vi "Encapsulate TCP Message.vi"(5 "source_id":u32, 7 "target_id":u32, 8 "error in (no error)":errorcluster, 9 "type_id":u32, 10 "Encapsulated Msg":refnum<class "Message.lvclass">) -> (0 "error out":errorcluster, 2 "TCP Payload":string)   [LabVIEW 2020, in "Vecto.lvlib"]
uses:
  Vecto.lvlib
  <vilib>/IlluminatedG/IG Protoc/LV-Proto/Message/Message.lvclass
  SequenceCountService/SequenceCountService.lvclass
  proto/TcpPayload/Data.ctl
  proto/TcpPayload/TcpPayload.lvlib
panel:
  in  "SequenceCountService":refnum<class "SequenceCountService.lvclass">
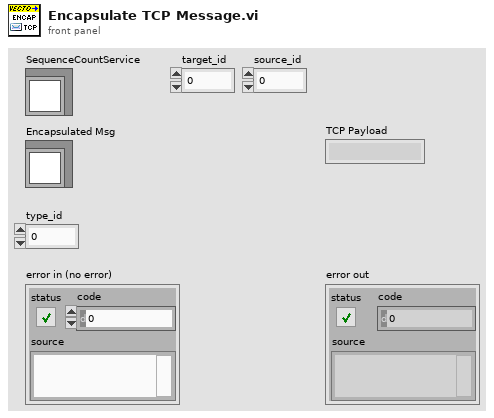
[diagram p1: front panel]
types:
  T1 = typedef "TcpPayload.lvlib/Data.ctl" = cluster{"target_node":u32, "target_task":u32, "source_id":u32, "sequence":u32, "timestamp":u64, "type_id":u32, "payload":u8[]}
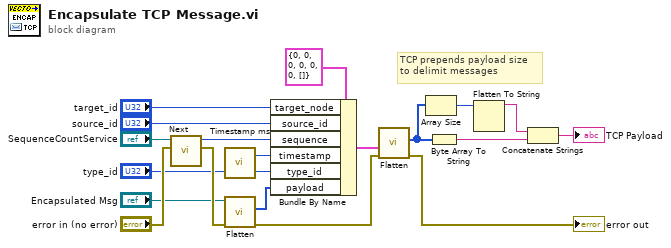
[diagram p0: block diagram]
diagram:
  # "TCP prepends payload size to delimit messages"
  n1 = call "Next.vi"("error in (no error)"="error in (no error)", "SequenceCountService in"="SequenceCountService") -> ("error out"=w18:errorcluster, "Sequence"=w9:u32)  [unwired: 8 in]
  n2 = call "Timestamp ms.vi"() -> ("Timestamp ms"=w11:u64)  [unwired: 7 in]
  n3 = call-dynamic "Flatten.vi"("error in (no error)"=w18, "Message in"="Encapsulated Msg") -> ("error out"=w7:errorcluster, "Buffer"=w12:u8[])  [unwired: 7 in, 1 out]
  n4 = Bundle By Name(cluster=T1 {"target_node"=0, "target_task"=0, "source_id"=0, "sequence"=0, "timestamp"=0, "type_id"=0, "payload"=[]} ("TcpPayload"), "target_node"="target_id", "source_id"="source_id", "sequence"=w9, "timestamp"=w11, "type_id"="type_id", "payload"=w12) -> (w8:T1)
  n5 = call "Flatten.vi"("error in"=w7, "Data"=w8) -> ("error out"=→"error out":errorcluster, "Buffer"=w4:u8[])  [unwired: 8 in]
  n6 = Array Size(array=w4) -> (size(s)=w3:i32)
  n7 = Byte Array To String(unsigned byte array=w4) -> (string=w5:string)
  n8 = Flatten To String(anything=w3) -> (data string=w1:string)  [unwired: 3 in, 2 out]
  n9 = Concatenate Strings(w1, w5) -> (→"TCP Payload":string)
